vi "SSL_CTX_use_certificate_chain_file.vi"(8 "error in (no error)":errorcluster, 10 "Certificate Chain File":path=path "C:/Program Files (x86)/National Instruments/RT Images/nissl/18.0.0/ca-bundle.crt", 11 "SSL-Context in":refnum<class "SSL-Context.lvclass">) -> (0 "error out":errorcluster, 3 "SSL-Context out":refnum<class "SSL-Context.lvclass">)   [LabVIEW 2013, in "OpenSSL Socket.lvlib" / "SSL-Context.lvclass"]
uses:
  SSL-Context.lvclass
  SSL-Lib/SSL-Lib.lvclass/SSL-Lib.ctl
  SSL-Context.lvclass/SSL-Context.ctl
  SSL-Lib/Read SSL Library Path.vi
  Read Handle.vi
  SSL-Lib/SSL-Lib.lvclass
panel:
  out "return type":i32
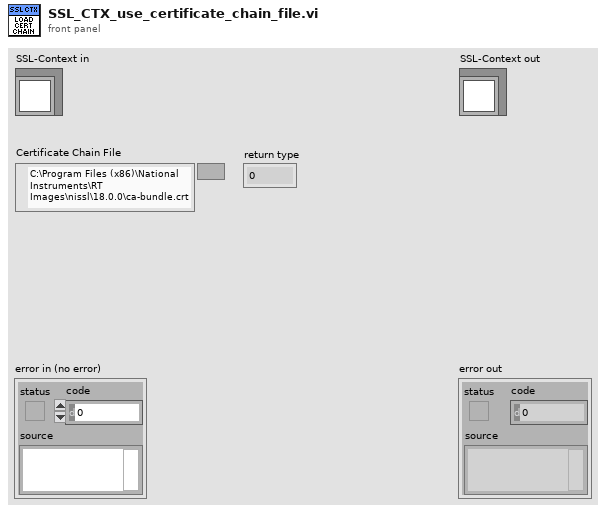
[diagram p1: front panel]
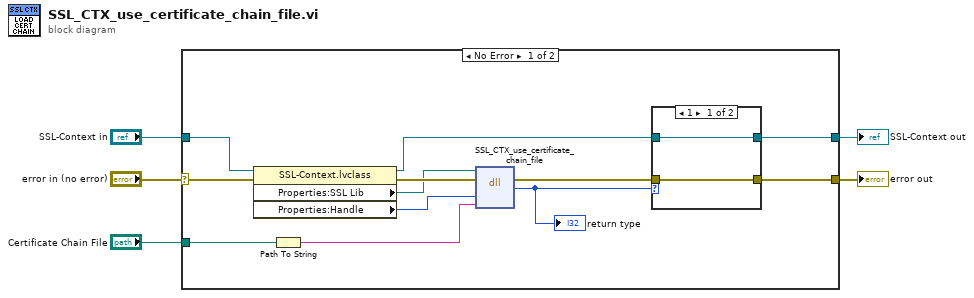
[diagram p0: block diagram]
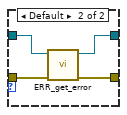
[diagram p2: hidden frame]
diagram:
  n1 = case shown="No Error" "error in (no error)" {
    selector: "error in (no error)" -> [w17 w25]
    tunnel: [w9 w25] -> w4
    tunnel: [w10 w24] -> w2
    tunnel: "SSL-Context in" -> [w15 w24]
    tunnel: "Certificate Chain File" -> [w7 _]
    frame No Error {
      n2 = property class="SSL-Context.lvclass"(reference=w15, error in=w17) -> (reference out=w11:refnum<class "SSL-Context.lvclass">, error out=w16:errorcluster, "Properties:SSL Lib"=w14:path, "Properties:Handle"=w13:u64)
      n3 = Path To String(path=w7) -> (string=w6:string)
      n4 = dll-call lib="C:/Program Files (x86)/National Instruments/Shared/nissl/NIssleay32.dll" fn="SSL_CTX_use_certificate_chain_file"(path in=w14, error in=w16, "SSL_CTX"=w13, "file"=w6) -> (error out=w12:errorcluster, "return type"=w8:i32)  [unwired: 3 in, 1 out]
      "return type" <- w8
      n5 = case shown="1" w8 {
        tunnel: w12 -> [w19 w23]
        tunnel: w11 -> [w18 w22]
        tunnel: [w18 w21] -> w10
        tunnel: [w19 w20] -> w9
        frame 1 {
        }
        frame Default {
          n6 = call "ERR_get_error.vi"("error in (no error)"=w23, "SSL-Lib in"=w22) -> ("error out"=w20:errorcluster, "SSL-Lib out"=w21:refnum<class "SSL-Context.lvclass">)  [unwired: 8 in]
        }
      }
    }
    frame Error {
    }
  }
  "error out" <- w4
  "SSL-Context out" <- w2
